vi "createNewFile.vi"(8 "error in (no error)":errorcluster, 9 "isNewFilePathFromCounter":bool, 10 "filePath":path, 11 "Logger in":refnum<class "Logger.lvclass">) -> (0 "error out":errorcluster, 3 "Logger out":refnum<class "Logger.lvclass">)   [LabVIEW 2018, in "Logger.lvclass"]
doc: "Create the new log file. If the file path is \"/\", the internal file counter will be used to generate the new filename."
uses:
  Logger.lvclass
  Logger.lvclass/Logger.ctl
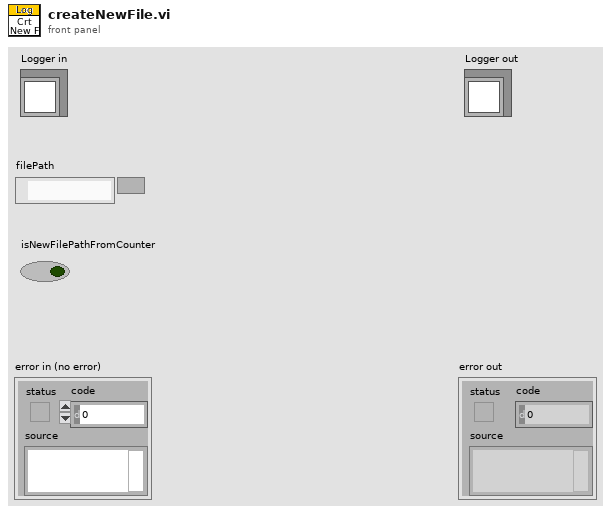
[diagram p1: front panel]
types:
  T1 = enum16{"open", "replace", "create", "open or create", "replace or create", "replace or create with confirmation"}
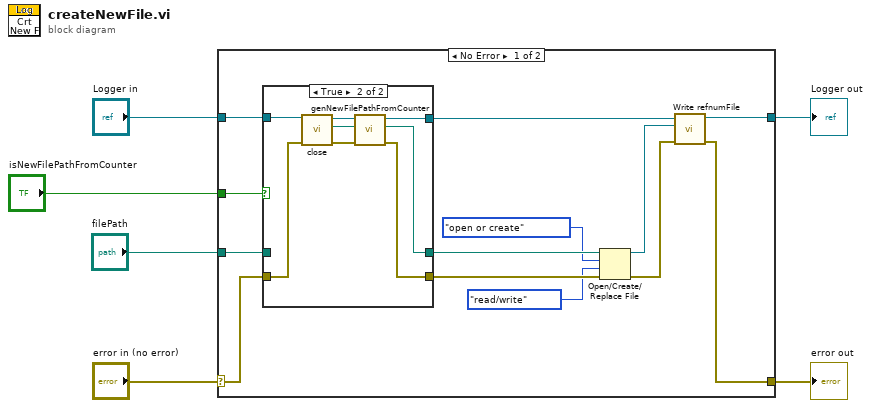
[diagram p0: block diagram]
diagram:
  n1 = case shown="No Error" "error in (no error)" {
    selector: "error in (no error)" -> [w17 w32]
    tunnel: [w7 w32] -> w5
    tunnel: [w10 w31] -> w3
    tunnel: "Logger in" -> [w16 w31]
    tunnel: "isNewFilePathFromCounter" -> [w19 _]
    tunnel: "filePath" -> [w18 _]
    frame No Error {
      n2 = case shown="True" w19 {
        tunnel: w18 -> [w22 _]
        tunnel: [w22 w28] -> w15
        tunnel: w17 -> [w20 w23]
        tunnel: w16 -> [w21 w27]
        tunnel: [w21 w30] -> w11
        tunnel: [w20 w29] -> w13
        frame False {
        }
        frame True {
          n3 = call "close.vi"("error in (no error)"=w23, "Logger in"=w27) -> ("error out"=w24:errorcluster, "filePathClosed"=w25:path, "Logger out"=w26:refnum<class "Logger.lvclass">)  [unwired: 7 in]
          n4 = call "genNewFilePathFromCounter.vi"("error in (no error)"=w24, "filePathOld"=w25, "Logger in"=w26) -> ("error out"=w29:errorcluster, "filePathNew"=w28:path, "Logger out"=w30:refnum<class "Logger.lvclass">)  [unwired: 6 in]
        }
      }
      n5 = Open/Create/Replace File(file path (use dialog)=w15, error in=w13, operation (0:open)=T1."open or create", access (0:read/write)=enum16{"read/write", "read-only", "write-only"}."read/write") -> (refnum out=w9:refnum<file>, error out=w8:errorcluster)  [unwired: 2 in, 1 out]
      n6 = call "Write refnumFile.vi"("error in (no error)"=w8, "refnumFile"=w9, "Logger in"=w11) -> ("error out"=w7:errorcluster, "Logger out"=w10:refnum<class "Logger.lvclass">)  [unwired: 7 in]
    }
    frame Error {
    }
  }
  "error out" <- w5
  "Logger out" <- w3
